vi "Drawbridge Reset.vi"(10 "Start?":bool) -> ()   [LabVIEW 2019]
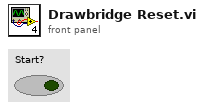
[diagram p1: front panel]
types:
  T1 = typedef "WPI_DigitalInputDevRef.ctl" = cluster{"DevStatus":errorcluster, "DIO Channel":T2}
  T2 = typedef "FPGA_DIOChannel.ctl" = enum8{"DIO 0", "DIO 1", "DIO 2", "DIO 3", "DIO 4", "DIO 5", "DIO 6", "DIO 7", "DIO 8", "DIO 9", "DIO MXP 0", "DIO MXP 1", "DIO MXP 2", "DIO MXP 3", "DIO MXP 4", "DIO MXP 5", "DIO MXP 6", "DIO MXP 7", "DIO MXP 8", "DIO MXP 9", "DIO MXP 10", "DIO MXP 11", "DIO MXP 12", "DIO MXP 13", "DIO MXP 14", "DIO MXP 15", "SPI Port CS1", "SPI Port CS2", "SPI Port CS3", "SPI Port MISO", "SPI Port MOSI", "Invalid"}
  T3 = typedef "WPI_MotorControlDeviceRef.ctl" = cluster{"DeviceStatus":errorcluster, "Type":T4, "PWM":cluster{"PWM Channel":T5, "DeadBand":T6}, "CAN":cluster{"Device Number":u8, "SetOutput VI Ref":variant, "GetOutput VI Ref":variant, "Enable VI Ref":variant, "Disable VI Ref":variant, "Data":variant}, "Invert":bool, "DIO PWM":cluster{"PWM \"Enable\" Channel":T5, "DIOChannel":T2, "PWM Rate":dbl}}
  T4 = typedef "WPI_MotorControlType.ctl" = enum16{"PWM", "CAN", "DIO PWM"}
  T5 = typedef "FPGA_DIOPWMChannel.ctl" = enum8{"PWM 0", "PWM 1", "PWM 2", "PWM 3", "PWM 4", "PWM 5", "PWM 6", "PWM 7", "PWM 8", "PWM 9", "PWM MXP 0", "PWM MXP 1", "PWM MXP 2", "PWM MXP 3", "PWM MXP 4", "PWM MXP 5", "PWM MXP 6", "PWM MXP 7", "PWM MXP 8", "PWM MXP 9", "Invalid"}
  T6 = typedef "WPI_PWMDeadband.ctl" = cluster{"Name":string, "maxPositivePwm":i32, "minPositivePwm":i32, "centerPwm":i32, "maxNegativePwm":i32, "minNegativePwm":i32, "angularRange":u16}
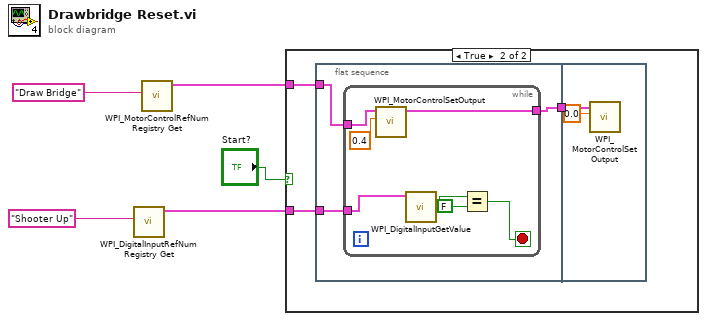
[diagram p0: block diagram]
diagram:
  n1 = call <vilib>:"WPI_DigitalInputRefNum Registry Get.vi"("refnum name"="Shooter Up") -> ("DigitalInputDevRef"=w1:T1)  [unwired: 9 in, 1 out]
  n2 = call <vilib>:"WPI_MotorControlRefNum Registry Get.vi"("refnum name"="Draw Bridge") -> ("MotorControlDevRef"=w2:T3)  [unwired: 9 in, 1 out]
  n3 = case shown="True" "Start?" {
    tunnel: w2 -> [_ w8]
    tunnel: w1 -> [_ w7]
    frame False {
    }
    frame True {
      n4 = flat-sequence {
        tunnel: w8 -> [w11]
        tunnel: w7 -> [w10]
        tunnel: [w9] -> w6
        tunnel: w6 -> [w20]
        frame #0 {
          n5 = while {
            tunnel: w11 -> [w18]
            tunnel: w10 -> [w16]
            tunnel: [w12] -> w9
            stop <- w13 stop-if-true
            n6 = call <vilib>:"WPI_MotorControlSetOutput.vi"("Output"=0.4, "MotorControlDevRef"=w18) -> ("MotorControlDevRef"=w12:T3)  [unwired: 7 in, 2 out]
            n7 = call <vilib>:"WPI_DigitalInputGetValue.vi"("DigitalInputDevRef"=w16) -> ("Value"=w15:bool)  [unwired: 8 in, 2 out]
            n8 = Equal?(x=w15, y=FALSE) -> (x = y?=w13:bool)
          }
        }
        frame #1 {
          n9 = call <vilib>:"WPI_MotorControlSetOutput.vi"("Output"=0.0, "MotorControlDevRef"=w20) -> ()  [unwired: 7 in, 3 out]
        }
      }
    }
  }
